vi "Elevator Mode Cycle.vi"(9 "Set to Auto":bool, 10 "Set to Safe":bool, 11 "Set to Manual":bool) -> (3 "Mode":T1)   [LabVIEW 2015]
uses:
  Common Code/Elevator Mode.ctl
  Robot Global Data.vi
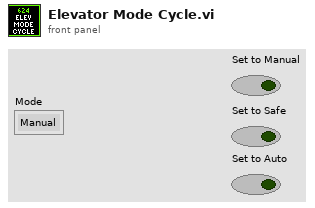
[diagram p1: front panel]
types:
  T1 = typedef "Elevator Mode.ctl" = enum16{"Manual", "Safe", "Auto"}
  T2 = enum16{"0", "1", "2", "3", "4", "5", "6", "7", "8", "9", "A", "B", "C", "D", "E", "F", "G", "H", "I", "J", "K", "L", "M", "N", "O", "P", "Q", "R", "S", "T", "U", "V", "W", "X", "Y", "Z", "F1", "F2", "F3", "F4", "F5", "F6", "F7", "F8", "F9", "F10", "F11", "F12", "F13", "F14", "F15", "ADD", "BACK", "BACKSLASH", "CAPITAL", "COMMA", "DECIMAL", "DELETE", "DIVIDE", "DOWN", "END", "EQUALS", "ESCAPE", "GRAVE (`)", "HOME", "INSERT", "LBRACKET", "LCONTROL", "LEFT", "L ALT", "LSHIFT", "LWIN", "MINUS", "MULTIPLY", "NEXT", "NUMLOCK", "NUMPAD_0", "NUMPAD_1", "NUMPAD_2", "NUMPAD_3", "NUMPAD_4", "NUMPAD_5", "NUMPAD_6", "NUMPAD_7", "NUMPAD_8", "NUMPAD_9", "PAUSE", "PERIOD", "PRIOR (PG UP)", "RBRACKET", "RCONTROL", "RETURN", "RIGHT", "R ALT", "RSHIFT", "RWIN", "SCROLL", "SEMICOLON", "SLASH", "SPACE", "SUBTRACT", "TAB", "UP", "ENTER (num pad)", "' (quote)"}
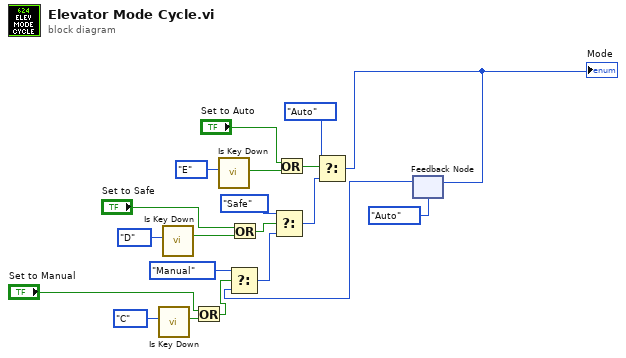
[diagram p0: block diagram]
diagram:
  n1 = call "Is Key Down.vi"("Key"=T2."C") -> ("Key Down?"=w3:bool)  [unwired: 10 in]
  n2 = call "Is Key Down.vi"("Key"=T2."D") -> ("Key Down?"=w6:bool)  [unwired: 10 in]
  n3 = Or(x="Set to Manual", y=w3) -> (x .or. y?=w4:bool)
  n4 = call "Is Key Down.vi"("Key"=T2."E") -> ("Key Down?"=w9:bool)  [unwired: 10 in]
  n5 = Or(x="Set to Safe", y=w6) -> (x .or. y?=w7:bool)
  n6 = Or(x="Set to Auto", y=w9) -> (x .or. y?=w10:bool)
  n7 = feedback #1(Elevator_Mode."Auto" ("Mode")) -> (w11:T1)
  n8 = Select(t=Elevator_Mode."Manual" ("Mode"), s=w4, f=w11) -> (s? t:f=w14:T1)
  n9 = Select(t=Elevator_Mode."Safe" ("Mode"), s=w7, f=w14) -> (s? t:f=w13:T1)
  n10 = Select(t=Elevator_Mode."Auto" ("Mode"), s=w10, f=w13) -> (s? t:f=w1:T1)
  "Mode" <- w1
  n11 = feedback-in #1(w1) -> ()
